vi "ClientNetworkInterface.vi"(0 "Server Port":u16=12500, 1 "Server Address":string="127.0.0.1") -> ()   [LabVIEW 2025]
uses:
  <vilib>/net/WFCN/Network Status.ctl
  ClientNetworkInterfaceGlobalVariables.vi
  <vilib>/net/WFCN/NI_WFCN.lvlib
panel:
  out "error out":errorcluster
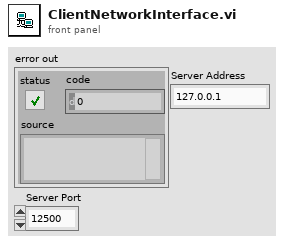
[diagram p1: front panel]
types:
  T1 = typedef "NI_WFCN.lvlib/Network Status.ctl" = enum16{"Indeterminate", "Configured", "Unconfigured"}
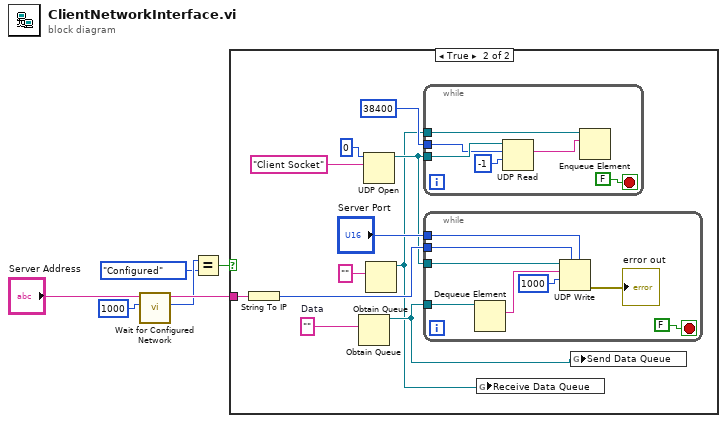
[diagram p0: block diagram]
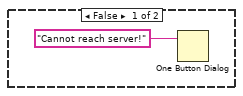
[diagram p2: hidden frame]
diagram:
  n1 = call <vilib>:"Wait for Configured Network.vi"("timeout in ms"=1000, "hostname or URL in"="Server Address") -> ("network status for remote host"=w3:T1, "hostname or URL out"=w5:string)  [unwired: 8 in]
  n2 = Equal?(x=w3, y=Network_Status."Configured" ("network status for remote host")) -> (x = y?=w4:bool)
  n3 = case shown="True" w4 {
    tunnel: w5 -> [_ w14]
    frame False {
      n4 = One Button Dialog(message="Cannot reach server!") -> ()  [unwired: 1 in, 1 out]
    }
    frame True {
      w17 = ""  # Data
      n5 = String To IP(1:w14) -> (0:w15:u32)
      n6 = Obtain Queue(element data type=w17) -> (queue out=w9:refnum<queue>)  [unwired: 4 in, 2 out]
      n7 = UDP Open(10:"Client Socket" ("service name"), 11:u16 0 ("port")) -> (port=w11:refnum<k16>)  [unwired: 3 in, 2 out]
      n8 = Obtain Queue(element data type="") -> (queue out=w8:refnum<queue>)  [unwired: 4 in, 2 out]
      n9 = while {
        tunnel: w8 -> [w32]
        tunnel: w11 -> [w28]
        tunnel: 38400 ("max size (548)") -> [w27]
        stop <- FALSE stop-if-true
        n10 = UDP Read(connection ID=w28, max size (548)=w27, timeout ms (25000)=-1) -> (data out=w31:string)  [unwired: 1 in, 4 out]
        n11 = Enqueue Element(queue=w32, element=w31) -> ()  [unwired: 2 in, 3 out]
      }
      n12 = while {
        tunnel: w9 -> [w26]
        tunnel: w15 -> [w23]
        tunnel: "Server Port" -> [w22]
        tunnel: w11 -> [w19]
        stop <- FALSE stop-if-true
        n13 = Dequeue Element(queue=w26) -> (element=w25:string)  [unwired: 2 in, 3 out]
        n14 = UDP Write(address=w23, port or service name=w22, connection ID=w19, data in=w25, 9:1000 ("timeout ms (25000)")) -> (error out=→"error out":errorcluster)  [unwired: 1 in, 1 out]
      }
      n15 = global write "ClientNetworkInterfaceGlobalVariables.vi" "Receive Data Queue"(w8) -> ()
      n16 = global write "ClientNetworkInterfaceGlobalVariables.vi" "Send Data Queue"(w9) -> ()
    }
  }
